vi "AlazarQueryCapability.vi"(0 "Handle":u64, 1 "Capability":u32(ring) items=["Get Serial Number"=268435492, "Get Latest Cal. Date"=268435494, "Get Latest Cal. Month"=268435501, "Get Latest Cal. Day"=268435502, "Get Latest Cal. Year"=268435503, "Memory Size"=268435498, "Board Type"=268435499, "ASOPC Type"=268435500, "Get PCIe Link Speed "=268435504, "Get PCIe Link Width"=268435505, "Get Max Pretrigger Samples"=268435526, "Get CPF Device"=268435569], 2 "error in (no error)":errorcluster) -> (3 "Handle":u64, 4 "Value":u32, 5 "Return Code":u32, 6 "error out":errorcluster)   [LabVIEW 2009]
doc: "Get a device attribute."
uses:
  ATSApi.dll
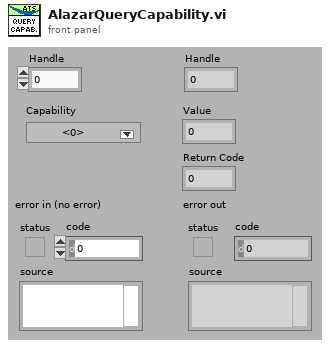
[diagram p1: front panel]
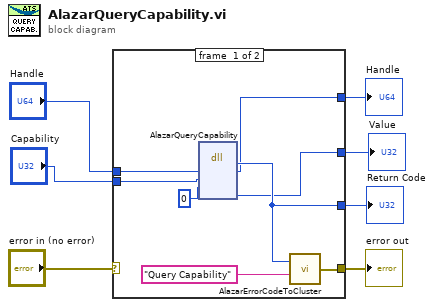
[diagram p0: block diagram]
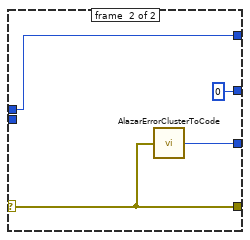
[diagram p2: hidden frame]
diagram:
  n1 = case shown="No Error" "error in (no error)" {
    selector: "error in (no error)" -> [_ w19]
    tunnel: [w12 w19] -> w6
    tunnel: [w14 w18] -> w5
    tunnel: "Handle" -> [w15 w17]
    tunnel: [w11 w17] -> w3
    tunnel: "Capability" -> [w10 _]
    tunnel: [w9 0] -> w1
    frame #0 {
      n2 = dll-call lib="ATSApi.dll" fn="AlazarQueryCapability"("handle"=w15, "capability"=w10, "reserved"=u32 0) -> ("return type"=w14:u32, "handle"=w11:u64, "value"=w9:u32)  [unwired: 6 in, 2 out]
      n3 = call "AlazarErrorCodeToCluster.vi"("Message"="Query Capability", "Error Code"=w14) -> ("error out"=w12:errorcluster)
    }
    frame #1 {
      n4 = call "AlazarErrorClusterToCode.vi"("error in (no error)"=w19) -> ("Error Code"=w18:u32)
    }
  }
  "Handle" <- w3
  "error out" <- w6
  "Return Code" <- w5
  "Value" <- w1
